vi "LabVIEW1.vi"() -> ()   [LabVIEW 2017]
panel:
  out "Tank":dbl(slide) scale=0.0..10.0
  in  "Dial":dbl(knob) scale=0.0..100.0
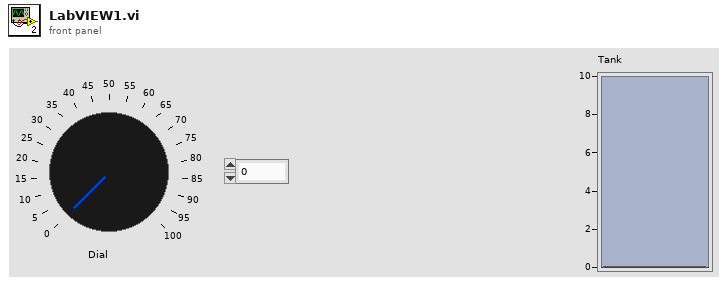
[diagram p1: front panel]
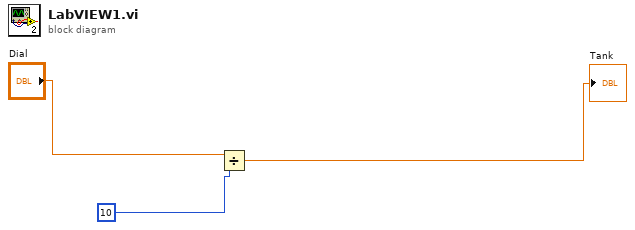
[diagram p0: block diagram]
diagram:
  n1 = Divide(x="Dial", y=10) -> (x/y=→"Tank":dbl)
